vi "Test B.vi"(6 "Station":T1(ring), 8 "error in (no error)":errorcluster) -> (0 "error out":errorcluster)   [LabVIEW 2019, in "Sequence Example.lvlib"]
uses:
  Sequence Example.lvlib
  400e6fd7-5c57-4563-98c8-4c487ac03ebd.vi
  d135eecd-02d8-4d26-94c7-1196041114e8.vi
  <vilib>/Utility/Data Type/Get Type Information.vi
  <vilib>/Utility/error.llb/Trim Whitespace.vi
  <vilib>/XXW Engineering/Test Bench Tools/Unit Test Engine Tools/Almost Equal.vi
  <vilib>/XXW Engineering/Test Bench Tools/Unit Test Engine Tools/Unit Test Engine Tools.lvlib
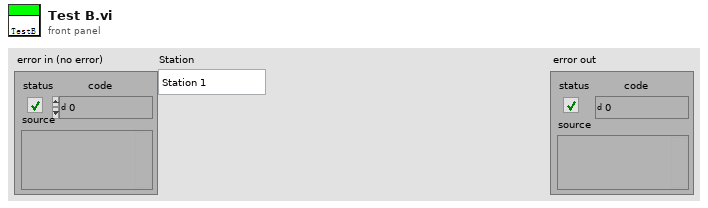
[diagram p1: front panel]
types:
  T1 = enum16{"Station 1", "Station 2", "Station 3", "Station 4"}
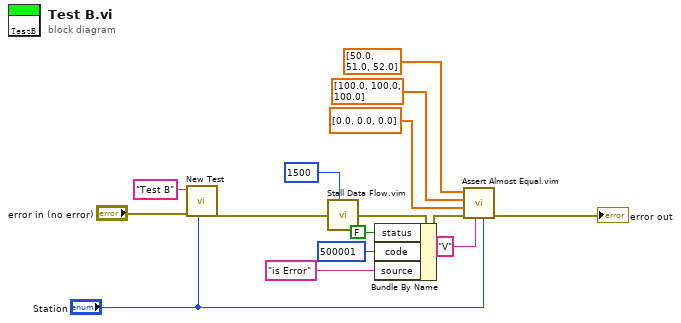
[diagram p0: block diagram]
diagram:
  n1 = call <vilib>:"New Test.vi"("Station"="Station", "error in (no error)"="error in (no error)", "Test"="Test B") -> ("error out"=w13:errorcluster)  [unwired: 8 in]
  n2 = call "Stall Data Flow.vim"("value in"=w13, "milliseconds to wait"=u32 1500) -> ("value out"=w9:errorcluster)  [unwired: 1 out]
  n3 = Bundle By Name(cluster=w9, "status"=FALSE, "code"=500001, "source"="is Error") -> (w4:errorcluster)
  n4 = call "Assert Almost Equal.vim"("Station"="Station", "Unit"="V", "error in (no error)"=w4, "Low limit"=dbl[] [0.0, 0.0, 0.0], "High limit"=dbl[] [100.0, 100.0, 100.0], "X"=dbl[] [50.0, 51.0, 52.0]) -> ("error out"=→"error out":errorcluster)  [unwired: 5 in]
